vi "ROI entry-Handle ROI change.vi"(8 "error in (no error)":errorcluster, 9 "Offsets cluster":T1, 11 "ROI management":T2) -> (0 "error out":errorcluster, 2 "No ROI":bool, 3 "Number of ROI":i32)   [LabVIEW 2013]
uses:
  Typedefs/ROI management FG states.ctl
  Typedefs/Offsets cluster.ctl
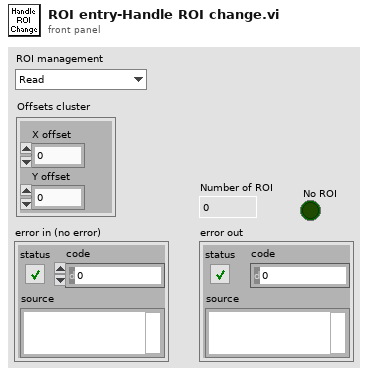
[diagram p1: front panel]
types:
  T1 = typedef "Offsets cluster.ctl" = cluster{"X offset":i8, "Y offset":i8}
  T2 = typedef "ROI management FG states.ctl" = enum16{"Read", "Write", "Clear Last", "Clear All", "Update ROIs time", "Reload last ROI set", "Offset all ROI", "Offset visible ROI"}
  T3 = typedef "ROI parameters data type.ctl" = cluster{"ROI index":dbl, "ROI ID":dbl, "ROI Time (ns)":dbl, "Pixels in ROI":dbl, "X start":dbl, "Y start":dbl, "Z start":dbl, "X stop":dbl, "Y stop":dbl, "Z stop":dbl, "Angle (deg)":dbl, "Composite ID":dbl, "Number of lines":dbl, "Frame Size":dbl, "Zoom":dbl, "Laser Power (%)":dbl, "ROI group ID":dbl}
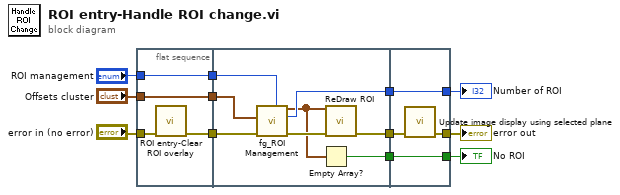
[diagram p0: block diagram]
diagram:
  n1 = flat-sequence {
    tunnel: [w16] -> w12
    tunnel: "error in (no error)" -> [w15]
    tunnel: [w14] -> w8
    tunnel: "ROI management" -> [w14]
    tunnel: "Offsets cluster" -> [w13]
    tunnel: [w13] -> w1
    tunnel: [w19] -> w11
    tunnel: w12 -> [w24]
    tunnel: w8 -> [w23]
    tunnel: [w22] -> w5
    tunnel: [w21] -> w4
    tunnel: w1 -> [w17]
    tunnel: [w25] -> w9
    tunnel: w11 -> [w26]
    tunnel: [w28] -> w6
    tunnel: w5 -> [w28]
    tunnel: [w27] -> w3
    tunnel: w4 -> [w27]
    frame #0 {
      n2 = call "ROI entry-Clear ROI overlay.vi"("error in (no error)"=w15) -> ("error out"=w16:errorcluster)  [unwired: 9 in, 1 out]
    }
    frame #1 {
      n3 = call "fg_ROI Management.vi"("Function"=w23, "error in (no error)"=w24, "Offsets cluster"=w17) -> ("error out"=w20:errorcluster, "Number of ROI"=w22:i32, "ROI Setup"=w18:T3[])  [unwired: 4 in, 2 out]
      n4 = Empty Array?(array=w18) -> (empty?=w21:bool)
      n5 = call "ReDraw ROI.vi"("error in"=w20, "XYZ Coordinates"=w18) -> ("error out"=w19:errorcluster)  [unwired: 9 in]
    }
    frame #2 {
      n6 = call "Update image display using selected plane.vi"("error in (no error)"=w26) -> ("error out"=w25:errorcluster)  [unwired: 10 in]
    }
  }
  "error out" <- w9
  "Number of ROI" <- w6
  "No ROI" <- w3
